vi "Report Core.vi"(8 "error in":errorcluster, 9 "Received":path, 10 "Approved":path, 11 "Report With LVCompare in":refnum<class "Report With LVCompare.lvclass">) -> (0 "error out":errorcluster, 2 "Worked?":bool, 3 "Report With LVCompare out":refnum<class "Report With LVCompare.lvclass">)   [LabVIEW 2020, in "Approval Tests.lvlib" / "Report With LVCompare.lvclass"]
uses:
  Report With LVCompare.lvclass
  Report With LVCompare.lvclass/Report With LVCompare.ctl
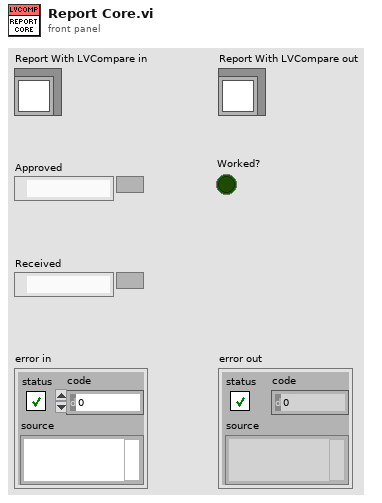
[diagram p1: front panel]
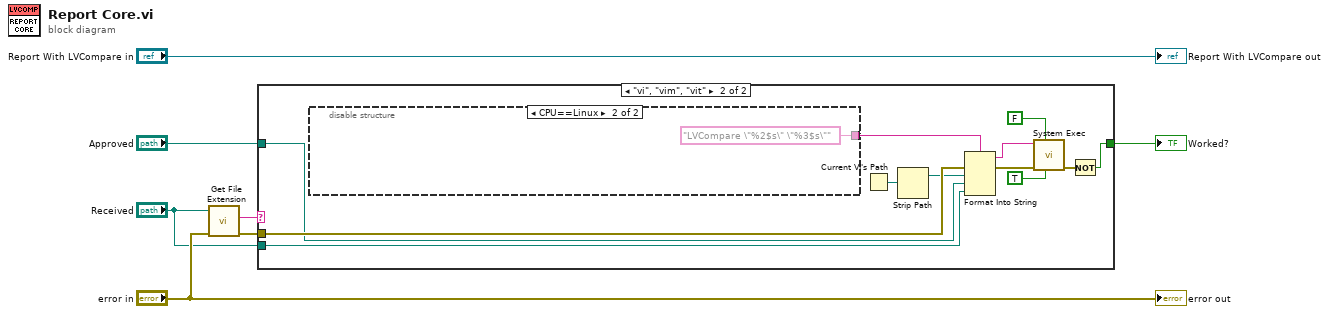
[diagram p0: block diagram]
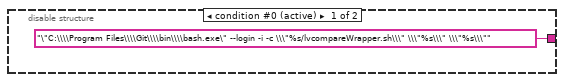
[diagram p3: hidden frame]
diagram:
  n1 = call <vilib>:"Get File Extension.vi"("error in (no error)"="error in", "file"="Received") -> ("error out"=w7:errorcluster, "lowercase file extension"=w4:string)  [unwired: 5 in, 3 out]
  n2 = case shown="\"vi\", \"vim\", \"vit\"" w4 {
    tunnel: w7 -> [_ w18]
    tunnel: [_ w16] -> w3
    tunnel: "Approved" -> [_ w10]
    tunnel: "Received" -> [_ w9]
    frame "False", Default {
    }
    frame "vi", "vim", "vit" {
      n3 = disable-structure shown="CPU==Linux" {
        disable-tunnel: ["\"C:\\\\Program Files\\\\Git\\\\bin\\\\bash.exe\" --login -i -c \\\"%s/lvcompareWrapper.sh\\\" \\\"%s\\\" \\\"%s\\\"" "LVCompare \"%2$s\" \"%3$s\""] -> w13
        frame condition #0 (active) {
        }
        frame condition #1 {
        }
      }
      n4 = Current VI's Path() -> (path=w12:path)
      n5 = Strip Path(path=w12) -> (stripped path=w11:path)  [unwired: 1 out]
      n6 = Format Into String(format string=w13, error in=w18, w11, w10, w9) -> (resulting string=w8:string, error out=w17:errorcluster)  [unwired: 1 in]
      n7 = call <vilib>:"System Exec.vi"("run minimized? (F)"=TRUE, "wait until completion? (T)"=FALSE, "error in (no error)"=w17, "command line"=w8) -> ("error out"=w19:errorcluster)  [unwired: 4 in, 3 out]
      n8 = Not(x=w19) -> (.not. x?=w16:bool)
    }
  }
  "Worked?" <- w3
  "error out" <- "error in"
  "Report With LVCompare out" <- "Report With LVCompare in"
